vi "Analog Gyro.vi"() -> ()   [LabVIEW 2025]
doc: "Analog Gyro Example\n\nThis VI shows how to use an analog gyro.\n\nThis example expects a USB cable connected from your development PC to the Type B USB Jack (next to the power input) on the roboRIO.\n\nThis example expects the Driver Station to be running."
uses:
  <vilib>/Rock Robotics/SystemInterfaces/AI/FPGA_AIGyroChannel.ctl
  <vilib>/Rock Robotics/WPI/Gyro/WPI_GyroAnalogOpen.vi
panel:
  out "Angle":dbl(knob) scale=0.0..360.0
  in  "Gain (VoltsPerDegree/Second)":dbl=0.007
  in  "stop":bool
  in  "Reset Zero Position":bool
  in  "Channel":T1
  # "Set these inputs before running."
  # "This can be set while running."
  # "This will display the current gyro angle."
  # "Analog Devices\nADW22307"
  # "Generic Gyro Wiring:\nroboRIO AI0 S (white wire) to gyro RATE\nroboRIO AI0 V (red wire) to gyro 5V\nroboRIO AI0     (black wire) to gyro GND"
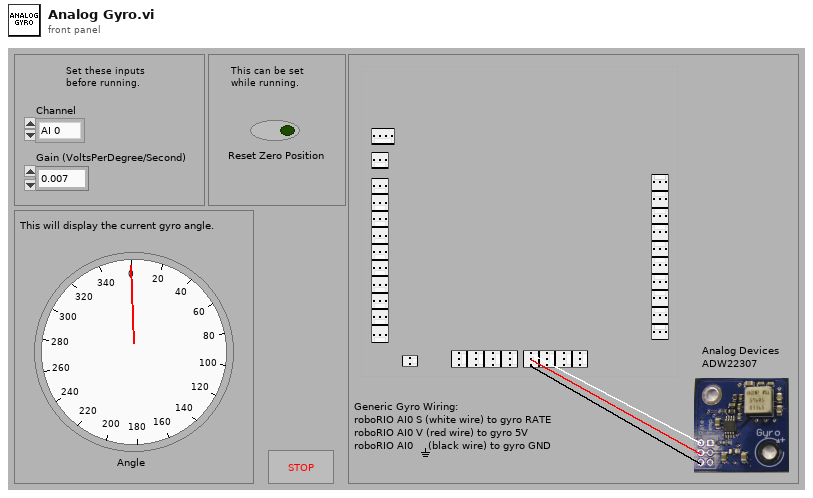
[diagram p1: front panel]
types:
  T1 = typedef "FPGA_AIGyroChannel.ctl" = enum8{"AI 0", "AI 1", "Invalid"}
  T2 = typedef "WPI_GyroDevRef.ctl" = cluster{"DevStatus":errorcluster, "Analog Channel":T3, "Gain (VoltsPerDegree/Second)":dbl, "Gyro Type":enum16{"Analog", "XRS450"}, "Handle":i32, "SPI Bus":T4, "Device Found":bool, "Sample Rate":dbl, "Calibrate On Open":bool, "Offset":dbl}
  T3 = typedef "FPGA_AIChannel.ctl" = enum8{"AI 0", "AI 1", "AI 2", "AI 3", "AI MXP 0", "AI MXP 1", "AI MXP 2", "AI MXP 3", "Invalid"}
  T4 = typedef "spi_bus.ctl" = enum16{"SPI On-Board, CS0", "SPI On-Board, CS1", "SPI On-Board, CS2", "SPI On-Board, CS3", "SPI MXP", "Invalid"}
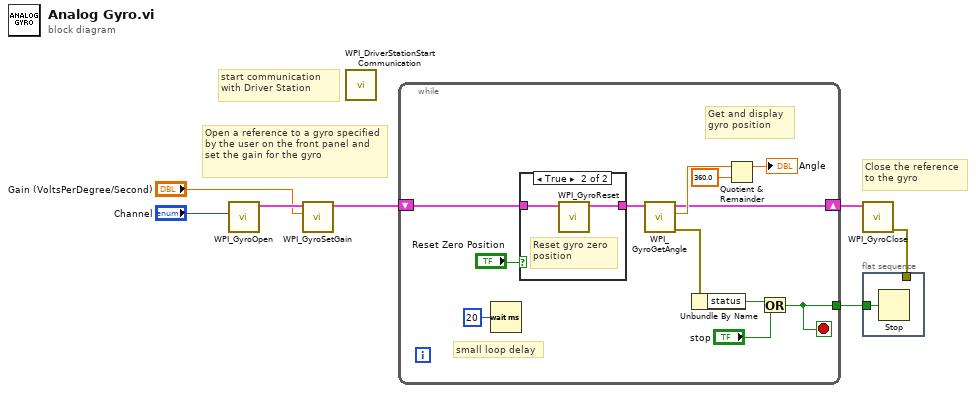
[diagram p0: block diagram]
diagram:
  # "start communication with Driver Station"
  # "Close the reference\nto the gyro"
  # "Open a reference to a gyro specified by the user on the front panel and set the gain for the gyro"
  n1 = call-poly <vilib>:"WPI_GyroOpen.vi"("Analog Channel"="Channel") -> ("GyroDevRef"=w6:T2)  [unwired: 8 in, 2 out]
  n2 = call <vilib>:"WPI_GyroSetGain.vi"("Gain (VoltsPerDegree/Second)"="Gain (VoltsPerDegree/Second)", "GyroDevRef"=w6) -> ("GyroDevRef"=w5:T2)  [unwired: 1 in, 8 out]
  n3 = call <vilib>:"WPI_DriverStationStart Communication.vi"() -> ()  [unwired: 3 in, 9 out]
  n4 = while {
    shift-right: [w15] -> w7
    shift-left: w5 -> [w18]
    tunnel: [w13] -> w2
    stop <- w13 stop-if-true
    # "small loop delay"
    # "Get and display\ngyro position"
    n5 = Wait (ms)(milliseconds to wait=u32 20) -> ()  [unwired: 1 out]
    n6 = case shown="True" "Reset Zero Position" {
      tunnel: w18 -> [w20 w22]
      tunnel: [w20 w21] -> w17
      frame False {
      }
      frame True {
        # "Reset gyro zero \nposition"
        n7 = call <vilib>:"WPI_GyroReset.vi"("GyroDevRef"=w22) -> ("GyroDevRef"=w21:T2)  [unwired: 10 out]
      }
    }
    n8 = call <vilib>:"WPI_GyroGetAngle.vi"("GyroDevRef"=w17) -> ("error out"=w10:errorcluster, "Angle"=w16:dbl, "GyroDevRef"=w15:T2)  [unwired: 1 in, 7 out]
    n9 = Unbundle By Name(w10) -> ("status"=w14:bool)
    n10 = Quotient & Remainder(x=w16, y=360.0) -> (x-y*floor(x/y)=→"Angle":dbl)  [unwired: 1 out]
    n11 = Or(x=w14, y="stop") -> (x .or. y?=w13:bool)
  }
  n12 = call <vilib>:"WPI_GyroClose.vi"("GyroDevRef"=w7) -> ("error out"=w1:errorcluster)  [unwired: 1 in, 9 out]
  n13 = flat-sequence {
    tunnel: w2 -> [w23]
    tunnel: w1 -> [_]
    frame #0 {
      n14 = Stop(stop? (T)=w23) -> ()
    }
  }
